vi "PAS_set_regulation_mode.vi"(8 "error in (no error)":errorcluster, 9 "MODE B":bool, 10 "MODE A":bool, 11 "VISA Refnum in":refnum<visa-resource-name>) -> (0 "error out":errorcluster, 1 "Success?":bool, 3 "VISA Refnum out":refnum<visa-resource-name>)   [LabVIEW 2020]
panel:
  out "read buffer":string
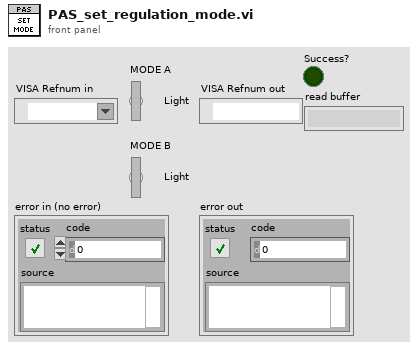
[diagram p1: front panel]
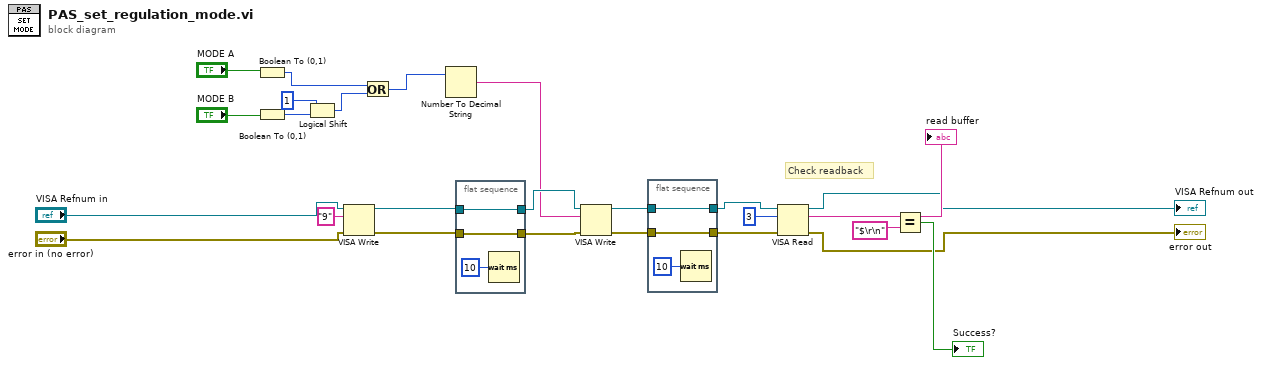
[diagram p0: block diagram]
diagram:
  # "Check readback"
  n1 = Boolean To (0,1)(Boolean="MODE A") -> (0, 1=w8:i16)
  n2 = Boolean To (0,1)(Boolean="MODE B") -> (0, 1=w11:i16)
  n3 = Logical Shift(y=i16 1, x=w11) -> (x << y=w9:i16)
  n4 = VISA Write(VISA resource name="VISA Refnum in", write buffer="9", error in (no error)="error in (no error)") -> (VISA resource name out=w20:refnum<visa-resource-name>, error out=w21:errorcluster)  [unwired: 1 out]
  n5 = Or(x=w8, y=w9) -> (x .or. y?=w7:i16)
  n6 = Number To Decimal String(number=w7) -> (decimal integer string=w18:string)  [unwired: 1 in]
  n7 = flat-sequence {
    tunnel: w20 -> [w27]
    tunnel: [w27] -> w22
    tunnel: w21 -> [w26]
    tunnel: [w26] -> w23
    frame #0 {
      n8 = Wait (ms)(milliseconds to wait=u32 10) -> ()  [unwired: 1 out]
    }
  }
  n9 = VISA Write(VISA resource name=w22, write buffer=w18, error in (no error)=w23) -> (VISA resource name out=w2:refnum<visa-resource-name>, error out=w4:errorcluster)  [unwired: 1 out]
  n10 = flat-sequence {
    tunnel: w2 -> [w30]
    tunnel: [w30] -> w1
    tunnel: w4 -> [w29]
    tunnel: [w29] -> w3
    frame #0 {
      n11 = Wait (ms)(milliseconds to wait=u32 10) -> ()  [unwired: 1 out]
    }
  }
  n12 = VISA Read(VISA resource name=w1, byte count=u32 3, error in (no error)=w3) -> (VISA resource name out=→"VISA Refnum out":refnum<visa-resource-name>, read buffer=w16:string, error out=→"error out":errorcluster)  [unwired: 1 out]
  "read buffer" <- w16
  n13 = Equal?(x=w16, y="$\r\n") -> (x = y?=→"Success?":bool)
